vi "Draw Tour.vi"(10 "Tour":u16[](array[numeric])=[1, 14, 13, 12, 7, 6, 15, 5, 11, 9, 10, 16, 3, 2, 4, 8, 1], 11 "Coordinate[]":T1[](array[typedef])=[{"x"=38.24, "y"=20.42}, {"x"=39.57, "y"=26.15}, {"x"=40.56, "y"=25.32}, {"x"=36.26, "y"=23.12}, {"x"=33.48, "y"=10.54}, {"x"=37.56, "y"=12.19}, {"x"=38.42, "y"=13.11}, {"x"=37.52, "y"=20.44}, {"x"=41.23, "y"=9.1}, {"x"=41.17, "y"=13.05}, {"x"=36.08, "y"=-5.21}, {"x"=38.47, "y"=15.13}, {"x"=38.15, "y"=15.35}, {"x"=37.51, "y"=15.17}, {"x"=35.49, "y"=14.32}, {"x"=39.36, "y"=19.56}]) -> (3 "City's":cluster{"X":dbl, "Y":dbl}[](graph))   [LabVIEW 2015, in "TSP Library.lvlib"]
uses:
  TSP Library.lvlib
  TypeDef/Coordinate.ctl
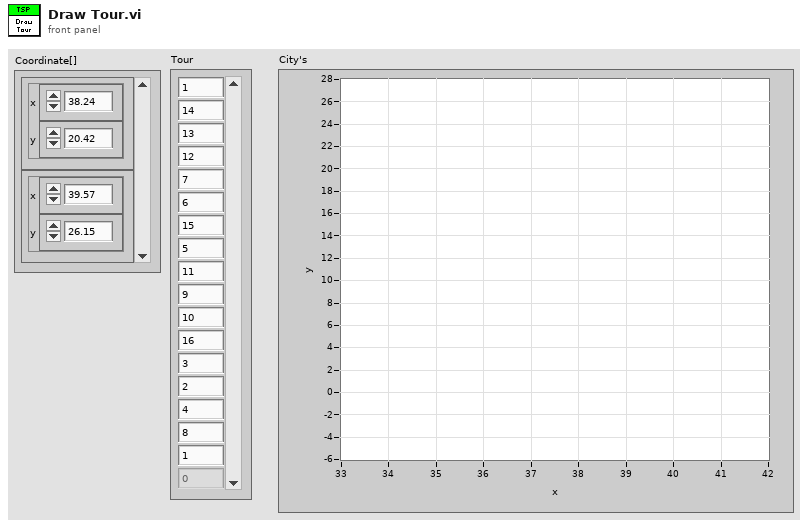
[diagram p1: front panel]
types:
  T1 = typedef "TSP Library.lvlib/Coordinate.ctl" = cluster{"x":dbl, "y":dbl}
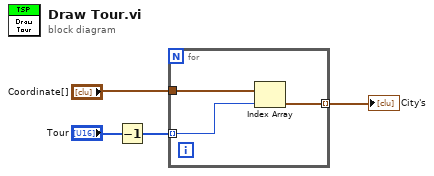
[diagram p0: block diagram]
diagram:
  n1 = Decrement(x="Tour") -> (x-1=w1:u16[])
  n2 = for {
    tunnel: "Coordinate[]" -> [w7]
    tunnel: w1 -> [w6] mode=indexing
    tunnel: [w5] -> w2 mode=indexing
    n3 = Index Array(array=w7, index=w6) -> (element=w5:T1)
  }
  "City's" <- w2
